vi "Que Ex - 2.vi"() -> ()   [LabVIEW 2022 SP3]
uses:
  <vilib>/ptbypt/NI_PtbyPt.lvlib
panel:
  out "Element in Que 2":i64
  out "Element in Que":i64
  in  "Que Time 2":u16(ring) items=["Same As Producer"=60, "Twice"=30, "1/2 the Prodcuer"=120]
  in  "Local Time":u16(ring) items=["Same As Producer"=60, "Twice"=30, "1/2 the Prodcuer"=120]
  in  "stop":bool
  out "Consumer with Que":dbl(graph)
  out "Consumer Local":dbl(graph)
  out "Producer":dbl(graph)
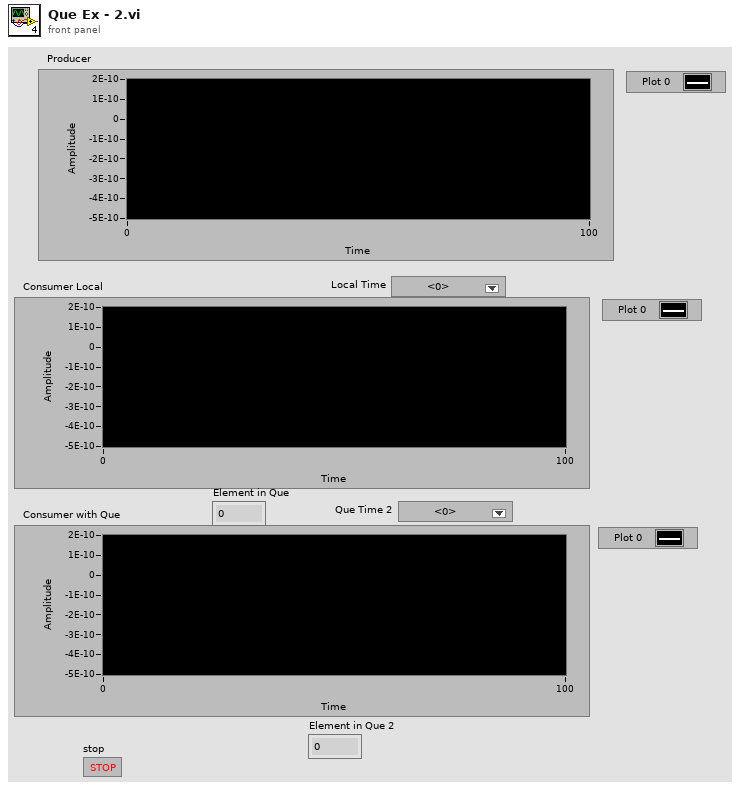
[diagram p1: front panel]
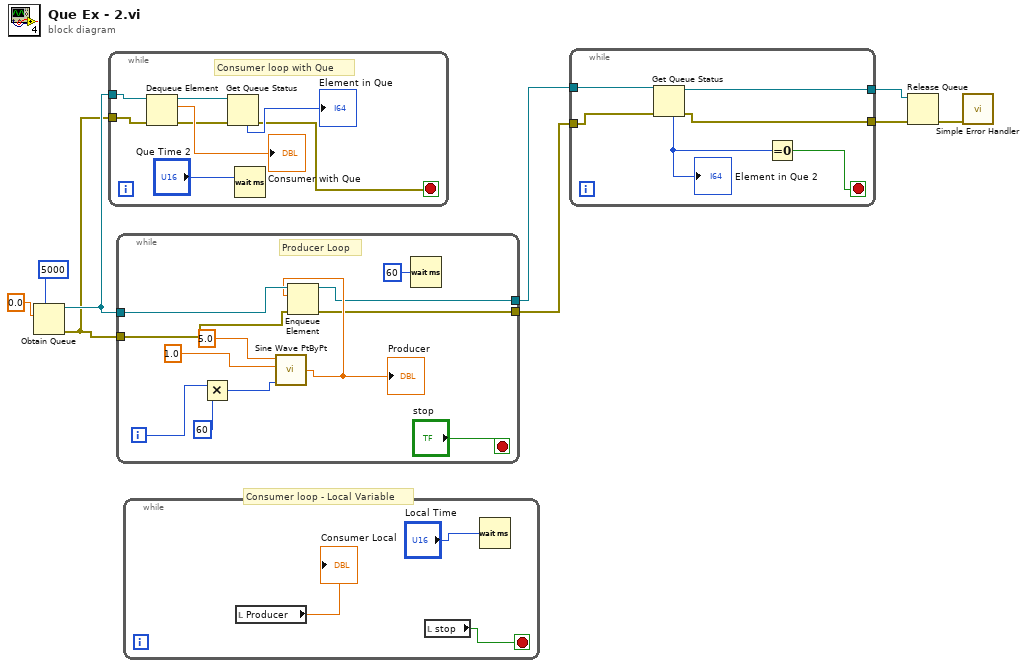
[diagram p0: block diagram]
diagram:
  # "Consumer loop - Local Variable"
  n1 = Obtain Queue(max queue size (-1, unlimited)=5000, element data type=0.0) -> (queue out=w7:refnum<queue>, error out=w6:errorcluster)  [unwired: 3 in, 1 out]
  n2 = while {
    tunnel: w7 -> [w16]
    tunnel: w6 -> [w15]
    stop <- w10 stop-if-true
    # "Consumer loop with Que"
    n3 = Dequeue Element(queue=w16, error in (no error)=w15) -> (queue out=w13:refnum<queue>, element=→"Consumer with Que":dbl, error out=w12:errorcluster)  [unwired: 1 in, 1 out]
    n4 = Get Queue Status(queue=w13, error in (no error)=w12) -> (error out=w10:errorcluster, # elements in queue=→"Element in Que":i32)  [unwired: 1 in, 6 out]
    n5 = Wait (ms)(milliseconds to wait="Que Time 2") -> ()  [unwired: 1 out]
  }
  n6 = while {
    tunnel: w7 -> [w22]
    tunnel: w6 -> [w21]
    tunnel: [w19] -> w5
    tunnel: [w18] -> w4
    i -> [w29]
    stop <- "stop" stop-if-true
    # "Producer Loop"
    n7 = Multiply(x=w29, y=60) -> (x*y=w25:i32)
    n8 = call <vilib>:"Sine Wave PtByPt.vi"("time"=w25, "frequency"=1.0, "amplitude"=5.0) -> ("sine wave"=w20:dbl)  [unwired: 1 in]
    "Producer" <- w20
    n9 = Enqueue Element(queue=w22, element=w20, error in (no error)=w21) -> (queue out=w19:refnum<queue>, error out=w18:errorcluster)  [unwired: 1 in, 1 out]
    n10 = Wait (ms)(milliseconds to wait=u32 60) -> ()  [unwired: 1 out]
  }
  n11 = while {
    stop <- w32 stop-if-true
    n12 = local read "Producer"() -> (→"Consumer Local":dbl)
    n13 = local read "stop"() -> (w32:bool)
    n14 = Wait (ms)(milliseconds to wait="Local Time") -> ()  [unwired: 1 out]
  }
  n15 = while {
    tunnel: w5 -> [w38]
    tunnel: w4 -> [w37]
    tunnel: [w36] -> w3
    tunnel: [w35] -> w2
    stop <- w33 stop-if-true
    n16 = Get Queue Status(queue=w38, error in (no error)=w37) -> (queue out=w36:refnum<queue>, error out=w35:errorcluster, # elements in queue=w34:i32)  [unwired: 1 in, 5 out]
    "Element in Que 2" <- w34
    n17 = Equal To 0?(x=w34) -> (x = 0?=w33:bool)
  }
  n18 = Release Queue(queue=w3, error in (no error)=w2) -> (error out=w1:errorcluster)  [unwired: 1 in, 2 out]
  n19 = call <vilib>:"Simple Error Handler.vi"("error in (no error)"=w1) -> ()  [unwired: 4 in, 5 out]
